vi "FromRepo.vi"(8 "error in":errorcluster, 9 "from repo cluster":T2, 10 "repository in":refnum<class "NISE_CEF_Repository.lvclass">, 11 "node in":refnum<class "RunTimeButton.lvclass">) -> (0 "error out":errorcluster, 2 "repository out":refnum<class "NISE_CEF_Repository.lvclass">, 3 "node":T1)   [LabVIEW 2015, in "RunTimeButton.lvclass"]
doc: "Grabs information from the Repo and stores it in the nodes."
uses:
  RunTimeButton.lvclass
  <vilib>/NI/Configuration Framework/Repository/NISE_CEF_Repository.lvclass
  <vilib>/NI/Configuration Framework/Node/FromRepoCluster.ctl
  <vilib>/NI/Configuration Framework/Node/NodeRef.ctl
  <vilib>/NI/Configuration Framework/Node/NISE_CEF_Node.lvclass
  CustomDeviceRepo/CustomDeviceRepo.lvclass
  Controls/RunTimeObjectsVariantCluster.ctl
  CustomDeviceRepo/CustomDeviceRepo.lvclass/CustomDeviceRepo.ctl
  RunTimeButton.lvclass/RunTimeButton.ctl
  CustomDeviceRepo/Read All Pages Properties.vi
  Write Button Properties.vi
  Configuration Tool.lvlib
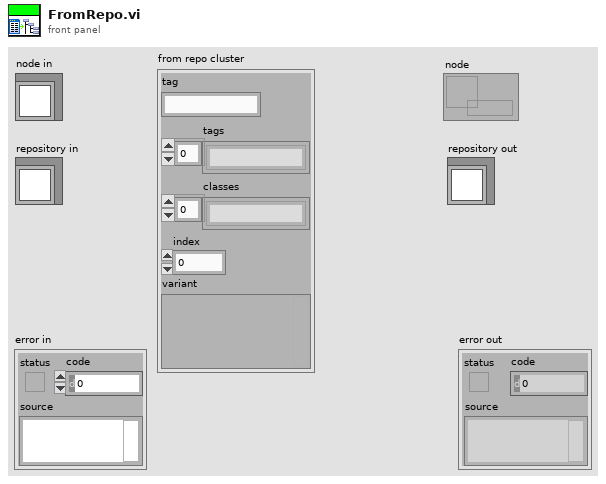
[diagram p1: front panel]
types:
  T1 = typedef "NISE_CEF_Node.lvclass/NodeRef.ctl" = refnum<data-value>
  T2 = typedef "NISE_CEF_Node.lvclass/FromRepoCluster.ctl" = cluster{"tag":string, "tags":string[], "classes":string[], "index":i32, "variant":variant}
  T3 = typedef "Configuration Tool.lvlib/RunTimeObjectsVariantCluster.ctl" = cluster{"Page Index":i32, "ActionVI Indexes":i32[]}
  T4 = typedef "Page Properties.ctl" = cluster{"Name":string, "Disallow Renaming":bool, "Delete Protection":bool, "Exlcude from Alphabetical order":bool, "Allow Multi-Selection":bool, "GUID":string, "Parent GUIDs":string[], "Glyph":T5, "Inactive Glyph":T5, "Broken Glyph":T5, "Item to Launch":T5, "Additional Information":string, "Copy":enum16{"copy", "disabled"}, "Paste":enum16{"Create", "CreatIfNotExists_GUID", "CreatIfNotExists_Name", "Replace", "Dialog"}, "Help":T6}
  T5 = typedef "Path Cluster.ctl" = cluster{"Path":path, "Path Type":enum16{"Absolute", "To Base", "To Common Doc Dir", "To Application Data Dir"}}
  T6 = typedef "help.ctl" = cluster{"Item to Launch":T5, "Section":string, "File Type":enum16{"chm", "other"}}
  T7 = typedef "ActionVIs Properties.ctl" = cluster{"Action VI On Delete":T5, "Action VI On Load":T5, "Action VI On Paste":T5, "Action VI On Target Type Change":T5, "Action VI On Delete Request":T5, "Action VI On Compile":T5, "Action VI On System Shutdown":T5, "Action VI On Save":T5, "Action VI On Download":T5}
  T8 = typedef "ButtonLists Properties.ctl" = cluster{"ID":string, "Glyph":T5, "Button Type":T9, "Referenced GUID":string, "Button Text":string, "Caption":string, "Tip Strip":string, "Documentation":string, "Dependency":T10}
  T9 = typedef "Button Type.ctl" = enum16{"Action", "Dialog", "Page", "Notification", "Separator"}
  T10 = typedef "Dependency three item small.ctl" = cluster{"File Path Control":path, "Path Type":enum16{"Absolute", "To Base", "To Common Doc Dir", "To Application Data Dir"}, "Behavior":enum16{"Static", "Dynamic"}}
  T11 = typedef "RunTimeMenus Properties.ctl" = cluster{"GUID":string, "Execution":T12, "MinNrOfChilds":u32, "Name":string, "Item to Launch":T5, "Dependency":T10, "Custom Population":T5, "Menu Item Type":enum16{"Action", "VI", "Separator", "Custom"}, "Behavior":enum16{"Nothing", "Open Front Panel"}, "Position":enum16{"Centered", "Mouse Pointer"}}
  T12 = typedef "Execution Types.ctl" = enum16{"silent", "modal", "floating", "default"}
  T13 = cluster{"General Page Properties":T4, "ActionVIs Properties":T7, "Button List Properties":T8[], "RunTime Menus Properties":T11[]}[]
  T14 = cluster{"General Page Properties":T4, "ActionVIs Properties":T7, "Button List Properties":T8[], "RunTime Menus Properties":T11[]}
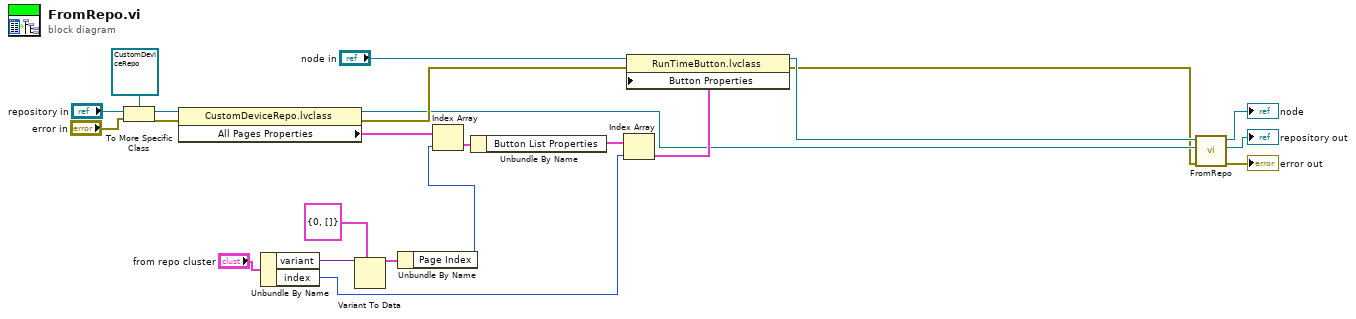
[diagram p0: block diagram]
diagram:
  n1 = To More Specific Class(target class=refnum<class "CustomDeviceRepo.lvclass"> refnum, reference="repository in", error in="error in") -> (specific class reference=w19:refnum<class "CustomDeviceRepo.lvclass">, error out=w20:errorcluster)
  n2 = property class="CustomDeviceRepo.lvclass"(reference=w19, error in=w20) -> (reference out=w5:refnum<class "CustomDeviceRepo.lvclass">, error out=w7:errorcluster, "All Pages Properties"=w13:T13)
  n3 = Unbundle By Name("from repo cluster") -> ("variant"=w14:variant, "index"=w9:i32)
  n4 = Variant To Data(type=T3 {"Page Index"=0, "ActionVI Indexes"=[]}, Variant=w14) -> (data=w2:T3)  [unwired: 1 in, 1 out]
  n5 = Unbundle By Name(w2) -> ("Page Index"=w1:i32)
  n6 = Index Array(array=w13, index=w1) -> (element=w11:T14)
  n7 = Unbundle By Name(w11) -> ("Button List Properties"=w10:T8[])
  n8 = Index Array(array=w10, index=w9) -> (element=w8:T8)
  n9 = property class="RunTimeButton.lvclass"(reference="node in", error in=w7, "Button Properties"=w8) -> (reference out=w6:refnum<class "RunTimeButton.lvclass">, error out=w4:errorcluster)
  n10 = call-parent "FromRepo.vi"("error in"=w4, "repository in"=w5, "node in"=w6) -> ("error out"=→"error out":errorcluster, "repository out"=→"repository out":refnum<class "NISE_CEF_Repository.lvclass">, "node"=→"node":T1)  [unwired: 6 in]
